vi "AWG_5421_Init_Session.vi"(8 "error in (no error)":errorcluster, 9 "EXCIT Inputs":T1={"Number of Excitations"=1, "Script Text"="", "Table of Waveforms"=[]} {"Number of Excitations" min=1 max=10}, 10 "AWG 5421 Inputs":T2={"Resource Name"="Waveform", "Sample Rate"=2000000.0, "Trigger Type"=2, "Trigger Source"="PFI0", "Waveform Gain"=0.31, "Digital Filter ON"=TRUE} {"Sample Rate" format="%.2p"; "Trigger Type" items=["None", "Software Edge", "Digital Edge", "Digital Level"]}, 11 "Use Software Trigger":bool) -> (0 "error out":errorcluster, 3 "Instrument handle out":refnum<k15>)   [LabVIEW 2024]
doc: "This VI inits a waveform generation session for AWG-5421. This is a basic example that shows how to setup the board in order to generate waveforms according to a script. \nBy default this configuration uses one channel CH0, and one script trigger ScriptTrigger0. The ScriptTrigger0 is waiting for an external trigger : i.e. a digital Edge on pin PFI 0 by default.\n\nThere are various options for the script to be used. Consult the Script control help for more information on configuring the example for specific scripts."
uses:
  controls/AWG_5421_Inputs.ctl
  <instrlib>/niFgen/niFgen.llb/niFgen_ctl Trigger Source Values (Ring).ctl
  controls/EXCIT_Inputs.ctl
  <instrlib>/niFgen/niFgen.llb/niFgen Output Mode.ctl
  <instrlib>/niFgen/niFgen.llb/niFgen_ctl Sample Clock Source Values (Ring).ctl
  <instrlib>/niFgen/niFgen.llb/niFgen Output Impedance.ctl
  <instrlib>/niFgen/niFgen.llb/niFgen_ctl Trigger Script - trigID Values (Ring).ctl
  <instrlib>/niFgen/niFgen.llb/niFgen_ctl Trigger DigEdge - Edge Values (Ring).ctl
  <instrlib>/niFgen/niFgen.llb/niFgen Configure Digital Edge Script Trigger.vi
  <instrlib>/niFgen/niFgen.llb/niFgen Configure Software Edge Script Trigger.vi
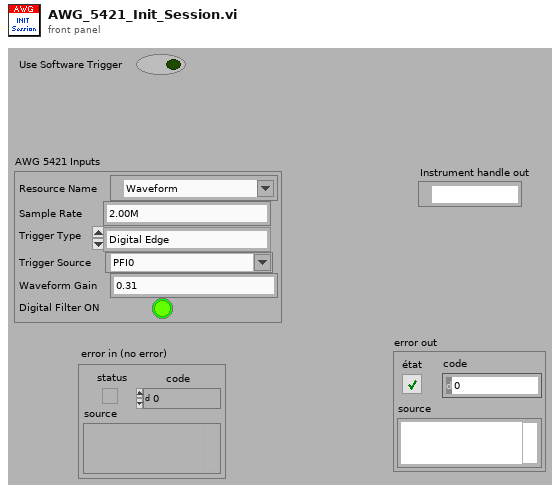
[diagram p1: front panel]
types:
  T1 = typedef "EXCIT_Inputs.ctl" = cluster{"Number of Excitations":i32, "Script Text":string, "Table of Waveforms":string[]}
  T2 = typedef "AWG_5421_Inputs.ctl" = cluster{"Resource Name":refnum<k15>, "Sample Rate":dbl, "Trigger Type":u16, "Trigger Source":T3, "Waveform Gain":dbl, "Digital Filter ON":bool}
  T3 = typedef "niFgen_ctl Trigger Source Values (Ring).ctl" = string
  T4 = typedef "niFgen_ctl Sample Clock Source Values (Ring).ctl" = string
  T5 = typedef "niFgen_ctl Trigger Script - trigID Values (Ring).ctl" = string
  T6 = typedef "niFgen Output Impedance.ctl" = i32
  T7 = typedef "niFgen Output Mode.ctl" = u32
  T8 = typedef "niFgen_ctl Trigger DigEdge - Edge Values (Ring).ctl" = i32
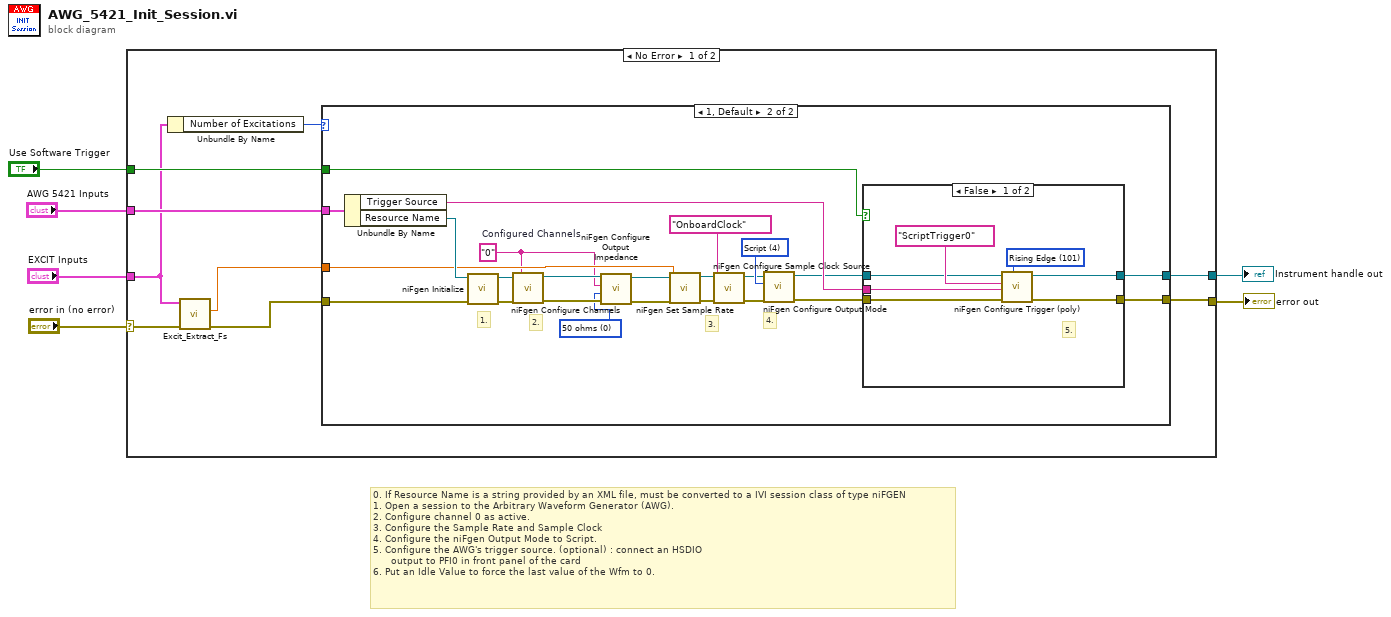
[diagram p0: block diagram]
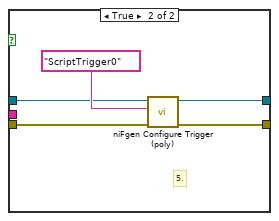
[diagram p3: hidden frame]
diagram:
  # "0. If Resource Name is a string provided by an XML file, must be converted to a IVI session class of type niFGEN\n1. Open a session to the Arbitrary Waveform Generator (AWG).\n2. Configure channel 0 as active. \n3. Configure the Sample Rate and Sample Clock\n4. Configure the niFgen Output Mode to Script.\n5. Configure the AWG's trigger source. (optional) : connect an HSDIO\n      output to PFI0 in front panel of the card \n6. Put an Idle Value to force the last value of the Wfm to 0."
  n1 = case shown="No Error" "error in (no error)" {
    selector: "error in (no error)" -> [w12 w53]
    tunnel: [w14 w53] -> w6
    tunnel: "AWG 5421 Inputs" -> [w9 _]
    tunnel: "Use Software Trigger" -> [w13 _]
    tunnel: [w15 _] -> w2
    tunnel: "EXCIT Inputs" -> [w8 _]
    frame No Error {
      n2 = Unbundle By Name(w8) -> ("Number of Excitations"=w7:i32)
      n3 = call "Excit_Extract_Fs.vi"("error in (no error)"=w12, "EXCIT Inputs"=w8) -> ("error out"=w11:errorcluster, "Sample Rate"=w10:dbl)  [unwired: 8 in]
      n4 = case shown="1, Default" w7 {
        tunnel: w9 -> [_ w40]
        tunnel: w11 -> [w16 w28]
        tunnel: [_ w27] -> w15
        tunnel: [w16 w26] -> w14
        tunnel: w13 -> [_ w25]
        tunnel: w10 -> [_ w24]
        frame 0 {
        }
        frame 1, Default {
          w21 = T6 0 items=["50 ohms", "75 ohms"] ("Impedance (default: 0=50 ohms)")
          w18 = "0"  # Configured Channels
          w38 = T7 4 items=["Standard Function", "Frequency List", "Arbitrary Waveform", "Arbitrary Sequence", "Script"] ("Output Mode")
          # "4."
          # "3."
          # "2."
          # "1."
          n5 = Unbundle By Name(w40) -> ("Trigger Source"=w30:T3, "Resource Name"=w29:refnum<k15>)
          n6 = call <instrlib>:"niFgen Initialize.vi"("error in (no error)"=w28, "Resource Name"=w29) -> ("error out"=w32:errorcluster, "Instrument Handle Out"=w33:refnum<k15>)  [unwired: 8 in]
          n7 = call <instrlib>:"niFgen Configure Channels.vi"("error in (no error)"=w32, "Channels"=w18, "Instrument Handle"=w33) -> ("error out"=w22:errorcluster, "Instrument Handle Out"=w23:refnum<k15>)  [unwired: 7 in]
          n8 = call <instrlib>:"niFgen Configure Output Impedance.vi"("error in (no error)"=w22, "Impedance (default: 0=50 ohms)"=w21, "Channel Name"=w18, "Instrument Handle"=w23) -> ("error out"=w20:errorcluster, "Instrument Handle Out"=w19:refnum<k15>)  [unwired: 6 in]
          n9 = call <instrlib>:"niFgen Set Sample Rate.vi"("error in (no error)"=w20, "Sample Rate (Samp/s)"=w24, "Instrument Handle"=w19) -> ("error out"=w34:errorcluster, "Instrument Handle Out"=w35:refnum<k15>)  [unwired: 7 in]
          n10 = call <instrlib>:"niFgen Configure Sample Clock Source.vi"("error in (no error)"=w34, "Source (Onboard Clock)"=T4 "OnboardClock", "Instrument Handle"=w35) -> ("error out"=w36:errorcluster, "Instrument Handle Out"=w37:refnum<k15>)  [unwired: 7 in]
          n11 = call <instrlib>:"niFgen Configure Output Mode.vi"("error in (no error)"=w36, "Output Mode (default: 0=Standard Function)"=w38, "Instrument Handle"=w37) -> ("error out"=w39:errorcluster, "Instrument Handle Out"=w17:refnum<k15>)  [unwired: 6 in]
          n12 = case shown="False" w25 {
            tunnel: w39 -> [w47 w52]
            tunnel: w30 -> [w42 _]
            tunnel: [w46 w51] -> w27
            tunnel: [w45 w50] -> w26
            tunnel: w17 -> [w41 w48]
            frame False {
              w43 = T8 101 items=["Rising Edge"=101, "Falling Edge"=102] ("Edge (Rising)")
              # "5."
              n13 = call-poly <instrlib>:"niFgen Configure Trigger (poly).vi"("Edge (Rising)"=w43, "error in (no error)"=w47, "Source"=w42, "Trigger ID (Script Trigger 0)"=T5 "ScriptTrigger0", "Instrument Handle"=w41) -> ("error out"=w45:errorcluster, "Instrument Handle Out"=w46:refnum<k15>)  [unwired: 5 in]
            }
            frame True {
              # "5."
              n14 = call-poly <instrlib>:"niFgen Configure Trigger (poly).vi"("error in (no error)"=w52, "Trigger ID (Script Trigger 0)"=T5 "ScriptTrigger0", "Instrument Handle"=w48) -> ("error out"=w50:errorcluster, "Instrument Handle Out"=w51:refnum<k15>)  [unwired: 7 in]
            }
          }
        }
      }
    }
    frame Error {
    }
  }
  "Instrument handle out" <- w2
  "error out" <- w6
